vi "Check Previous Error.vi"(8 "error in (no error)":errorcluster, 11 "VISA resource name in":refnum<visa-resource-name>) -> (0 "error out":errorcluster, 3 "VISA resource name":refnum<visa-resource-name>)   [LabVIEW 2022 SP3, in "CTI-Visa.lvlib"]
uses:
  <instrlib>/HandsOnPi2040/cti-drivers-lv-visa-main/CTI-Visa/CTI-Visa.lvlib
  <vilib>/Utility/error.llb/whitespace.ctl
  <vilib>/Utility/error.llb/Trim Whitespace One-Sided.vi
  <vilib>/Utility/error.llb/Error Cluster From Error Code.vi
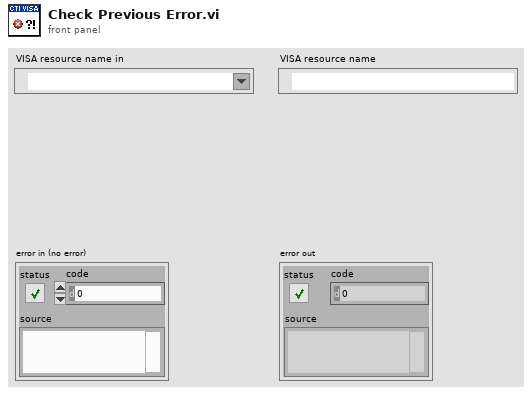
[diagram p1: front panel]
types:
  T1 = typedef "whitespace.ctl" = u16
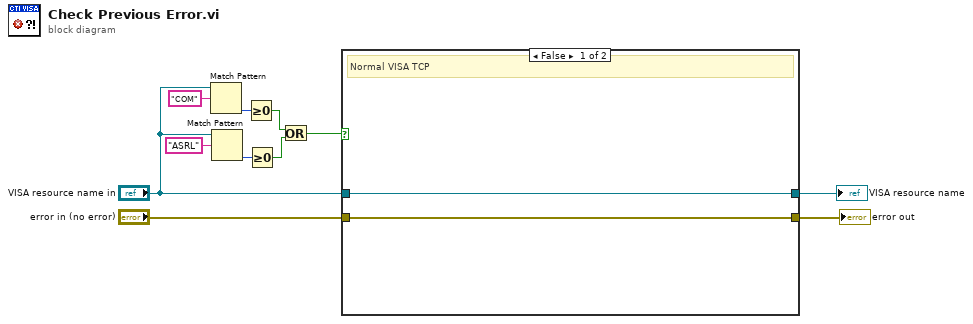
[diagram p0: block diagram]
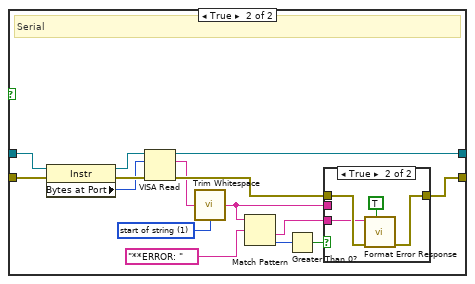
[diagram p2: hidden frame]
diagram:
  n1 = Match Pattern(string="VISA resource name in", regular expression="COM") -> (offset past match=w6:i32)  [unwired: 1 in, 3 out]
  n2 = Match Pattern(string="VISA resource name in", regular expression="ASRL") -> (offset past match=w5:i32)  [unwired: 1 in, 3 out]
  n3 = Greater Or Equal To 0?(x=w6) -> (x >= 0?=w4:bool)
  n4 = Greater Or Equal To 0?(x=w5) -> (x >= 0?=w3:bool)
  n5 = Or(x=w4, y=w3) -> (x .or. y?=w1:bool)
  n6 = case shown="False" w1 {
    tunnel: "error in (no error)" -> [w12 w26]
    tunnel: [w13 w23] -> w10
    tunnel: [w12 w15] -> w9
    tunnel: "VISA resource name in" -> [w13 w14]
    frame False {
      # "Normal VISA TCP"
    }
    frame True {
      w21 = T1 1 items=["both", "start of string", "end of string"] ("location (both)")
      # "Serial"
      n7 = property class="Instr"(reference=w14, error in=w26) -> (reference out=w25:refnum<visa-resource-name>, error out=w27:errorcluster, "Bytes at Port"=w24:u32)
      n8 = VISA Read(VISA resource name=w25, byte count=w24, error in (no error)=w27) -> (VISA resource name out=w23:refnum<visa-resource-name>, read buffer=w22:string, error out=w28:errorcluster)  [unwired: 1 out]
      n9 = call <vilib>:"Trim Whitespace.vi"("string"=w22, "location (both)"=w21) -> ("trimmed string"=w19:string)
      n10 = Match Pattern(string=w19, regular expression="**ERROR: " ("x")) -> (after substring=w18:string, offset past match=w17:i32)  [unwired: 1 in, 2 out]
      n11 = Greater Than 0?(x=w17) -> (x > 0?=w16:bool)
      n12 = case shown="True" w16 {
        tunnel: w28 -> [w29 w33]
        tunnel: w19 -> [_ _]
        tunnel: w18 -> [_ w32]
        tunnel: [w29 w30] -> w15
        frame False {
        }
        frame True {
          n13 = call <instrlib>:"Format Error Response.vi"("show call chain? (False)"=TRUE, "error in (no error)"=w33, "Error Response"=w32) -> ("error out"=w30:errorcluster)  [unwired: 8 in]
        }
      }
    }
  }
  "VISA resource name" <- w10
  "error out" <- w9
